vi "encodeStream.vi"(8 "error in (no error)":errorcluster, 11 "tBSONDouble in":refnum<class "tBSONDouble.lvclass">) -> (0 "error out":errorcluster, 2 "Byte Array":u8[](array[numeric]), 3 "tBSONDouble out":refnum<class "tBSONDouble.lvclass">)   [LabVIEW 2013, in "BSON.lvlib" / "tBSONDouble.lvclass"]
uses:
  tBSONDouble.lvclass
  tBSONElement/tBSONElement.lvclass
  getValue.vi
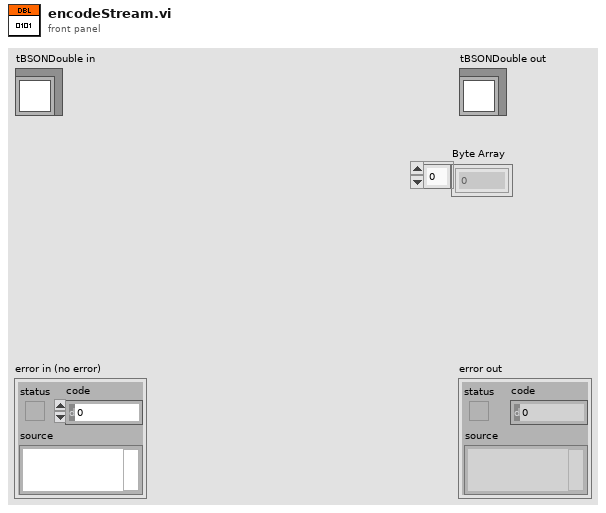
[diagram p1: front panel]
types:
  T1 = enum16{"big-endian, network order", "native, host order", "little-endian"}
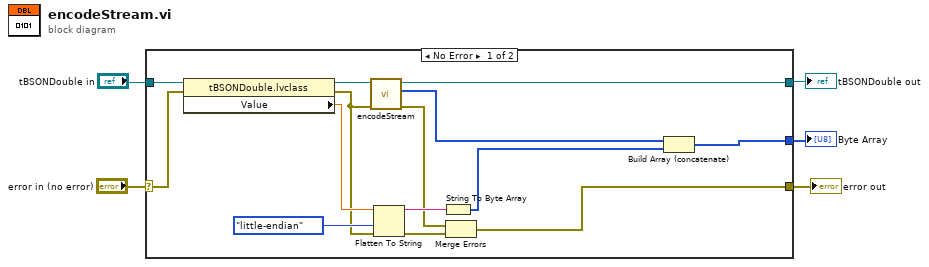
[diagram p0: block diagram]
diagram:
  n1 = case shown="No Error" "error in (no error)" {
    selector: "error in (no error)" -> [w19 w20]
    tunnel: "tBSONDouble in" -> [w16 w21]
    tunnel: [w6 w21] -> w4
    tunnel: [w17 w20] -> w2
    tunnel: [w18 _] -> w3
    frame No Error {
      n2 = property class="tBSONDouble.lvclass"(reference=w16, error in=w19) -> (reference out=w10:refnum<class "tBSONDouble.lvclass">, error out=w9:errorcluster, "Value"=w14:dbl)
      n3 = call-parent "encodeStream.vi"("error in (no error)"=w9, "tBSONElement in"=w10) -> ("error out"=w8:errorcluster, "Byte Array"=w7:u8[], "tBSONElement out"=w6:refnum<class "tBSONDouble.lvclass">)  [unwired: 7 in]
      n4 = Flatten To String(anything=w14, byte order (0:big-endian, network order)=T1."little-endian", error in (no error)=w9) -> (data string=w12:string, error out=w15:errorcluster)  [unwired: 1 in, 1 out]
      n5 = String To Byte Array(string=w12) -> (unsigned byte array=w11:u8[])
      n6 = Merge Errors(w8, w15) -> (w17:errorcluster)
      n7 = Build Array (concatenate)(w7, w11) -> (w18:u8[])
    }
    frame Error {
    }
  }
  "error out" <- w2
  "tBSONDouble out" <- w4
  "Byte Array" <- w3
